vi "stepper control.vi"(9 "error in (no error)":errorcluster, 10 "Distance to Travel (microns) \nup  is positive":dbl=250000.0, 11 "Velocity (microns/sec)":dbl=2500.0) -> (3 "error out":errorcluster)   [LabVIEW 2010]
uses:
  <vilib>/Instr/_visa.llb/VISA Configure Serial Port (Instr).vi
panel:
  out "return count":u32
  out "concatenated string":string
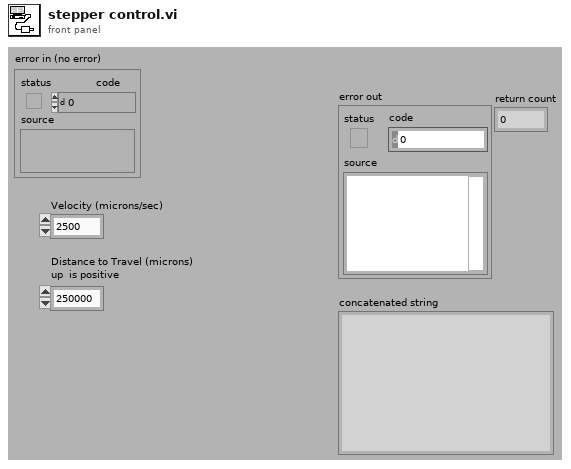
[diagram p1: front panel]
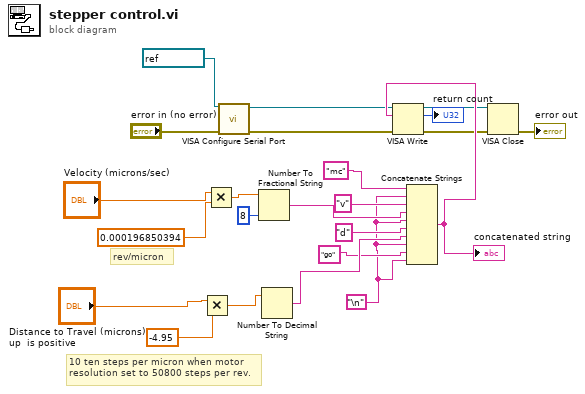
[diagram p0: block diagram]
diagram:
  w2 = "\n"
  # "10 ten steps per micron when motor\nresolution set to 50800 steps per rev."
  # "rev/micron"
  n1 = Multiply(x="Distance to Travel (microns) \nup  is positive", y=-4.95) -> (x*y=w18:dbl)
  n2 = Multiply(x="Velocity (microns/sec)", y=0.000196850394) -> (x*y=w23:dbl)
  n3 = call-poly "VISA Configure Serial Port"("VISA resource name"=refnum<visa-resource-name> "COM1", "error in (no error)"="error in (no error)") -> ("VISA resource name out"=w10:refnum<visa-resource-name>, "error out"=w8:errorcluster)  [unwired: 12 in]
  n4 = Number To Fractional String(number=w23, precision (6)=i16 8) -> (F-format string=w16:string)  [unwired: 2 in]
  n5 = Number To Decimal String(number=w18) -> (decimal integer string=w14:string)  [unwired: 1 in]
  n6 = Concatenate Strings("mc", w2, "v", w16, w2, "d", w14, w2, "go", w2) -> (w11:string)
  "concatenated string" <- w11
  n7 = VISA Write(VISA resource name=w10, write buffer=w11, error in (no error)=w8) -> (VISA resource name out=w7:refnum<visa-resource-name>, return count=→"return count":u32, error out=w6:errorcluster)
  n8 = VISA Close(VISA resource name=w7, error in (no error)=w6) -> (error out=→"error out":errorcluster)
